vi "Betonauswahl.vi"(8 "error in (no error)":errorcluster) -> (0 "error out":errorcluster)   [LabVIEW 2023]
doc: "Dieses VI ließt das config file für die Betonsorten und errechnet den Preis pro Menge .\nerstellt: Mate Zsolt Györfi\nDatum: 12.11.2025"
uses:
  <vilib>/Utility/miscctls.llb/LVRectTypeDef.ctl
  CONTROLS/fgv status.ctl
  CONTROLS/Betonauswahl_.ctl
panel:
  out "Preis":dbl
  in  "Betonauswahl":T1
  in  "Menge (m3)":dbl
  in  "Reserve Schalter 3":bool
  in  "Reserve Schalter 2":bool
  in  "Reserve Schalter":bool
  in  "Daten speichern":bool
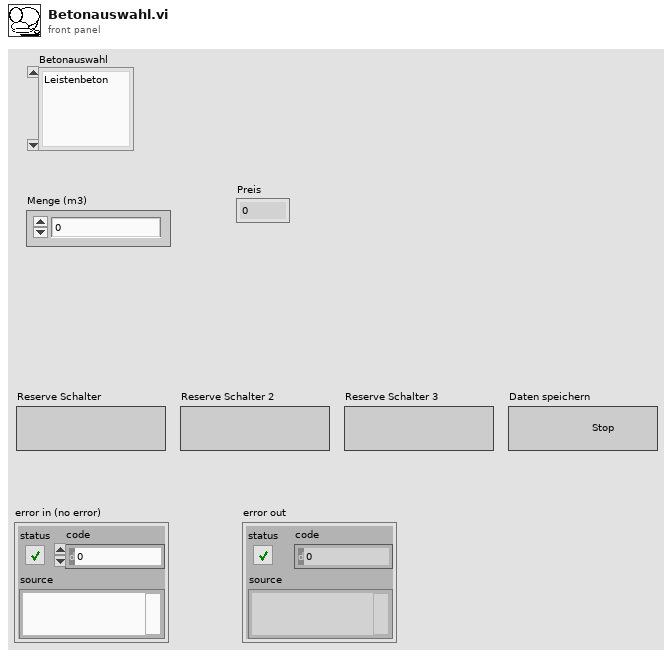
[diagram p1: front panel]
types:
  T1 = typedef "Betonauswahl_.ctl" = enum16{"Leistenbeton", "Erdfeuchter Beton", "Beton", "Erdfeuchter Starker Beton", "Starker Beton"}
  T2 = typedef "LVRectTypeDef.ctl" = cluster{"Left":i16, "Top":i16, "Right":i16, "Bottom":i16}
  T3 = typedef "fgv status.ctl" = enum16{"Read", "Write"}
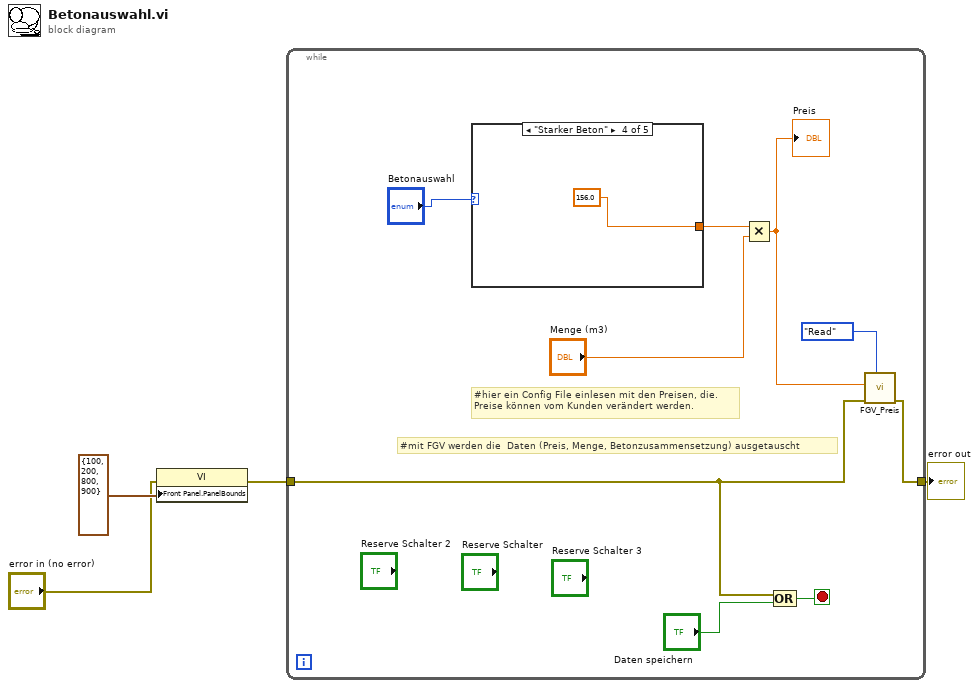
[diagram p0: block diagram]
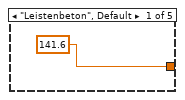
[diagram p2: hidden frame]
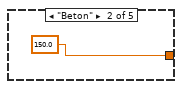
[diagram p3: hidden frame]
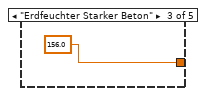
[diagram p4: hidden frame]
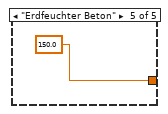
[diagram p5: hidden frame]
diagram:
  n1 = property class="VI"(error in="error in (no error)", "Front Panel.PanelBounds"=T2 {"Left"=100, "Top"=200, "Right"=800, "Bottom"=900} ("Front Panel Window:Panel Bounds")) -> (error out=w1:errorcluster)  [unwired: 1 in, 1 out]
  n2 = while {
    tunnel: [w7] -> w4
    tunnel: w1 -> [w8]
    stop <- w12 stop-if-true
    # "#mit FGV werden die  Daten (Preis, Menge, Betonzusammensetzung) ausgetauscht"
    # "#hier ein Config File einlesen mit den Preisen, die.\nPreise können vom Kunden verändert werden."
    n3 = case shown="\"Starker Beton\"" "Betonauswahl" {
      tunnel: [141.6 150.0 156.0 156.0 150.0] -> w10
      frame "Leistenbeton", Default {
      }
      frame "Beton" {
      }
      frame "Erdfeuchter Starker Beton" {
      }
      frame "Starker Beton" {
      }
      frame "Erdfeuchter Beton" {
      }
    }
    n4 = Multiply(x=w10, y="Menge (m3)") -> (x*y=w6:dbl)
    "Preis" <- w6
    n5 = Compound Arithmetic op=OR(w8, "Daten speichern") -> (w12:bool)
    n6 = call "FGV_Preis.vi"("FGV-Status"=fgv_status."Read", "error in (no error)"=w8, "Preis"=w6) -> ("error out"=w7:errorcluster)  [unwired: 7 in, 1 out]
  }
  "error out" <- w4
